vi "FTW-Collection-Construct-JSON.vi"(5 "Serialized Collection":string, 11 "error in":errorcluster) -> (4 "Collection":refnum<class "FTW-Collection.lvclass">, 6 "Valid Structure":bool, 15 "error out":errorcluster)   [LabVIEW 2012, in "FTW-Collection.lvclass"]
uses:
  FTW-Collection.lvclass
panel:
  # "Inputs"
  # "Outputs"
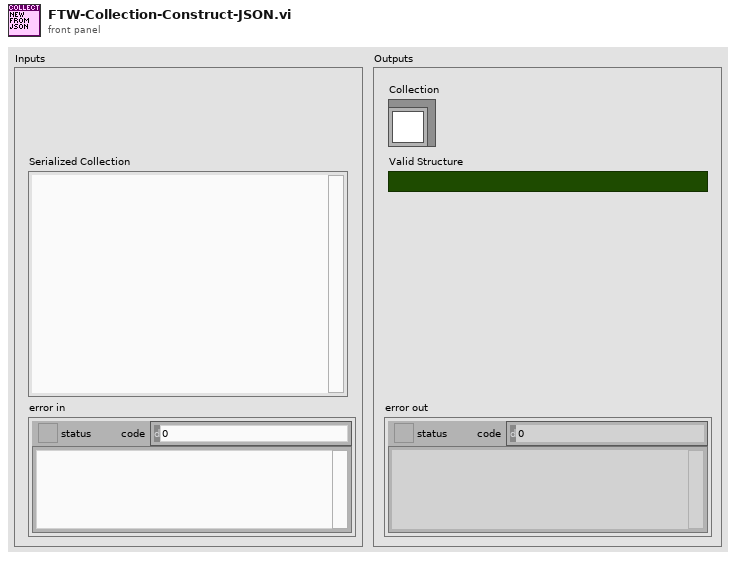
[diagram p1: front panel]
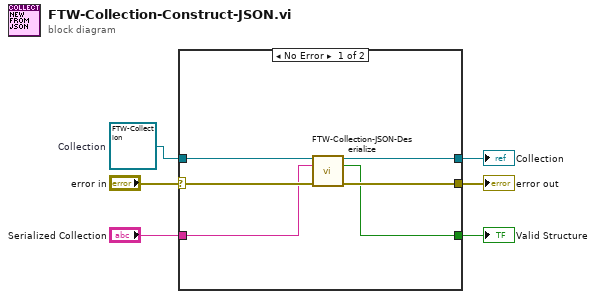
[diagram p0: block diagram]
diagram:
  w4 = refnum<class "FTW-Collection.lvclass"> refnum  # Collection
  n1 = case shown="No Error" "error in" {
    selector: "error in" -> [w11 w14]
    tunnel: [w9 w14] -> w6
    tunnel: w4 -> [w12 w13]
    tunnel: [w10 w13] -> w3
    tunnel: "Serialized Collection" -> [w8 _]
    tunnel: [w7 _] -> w1
    frame No Error {
      n2 = call "FTW-Collection-JSON-Deserialize.vi"("Collection"=w12, "Serialized Collection"=w8, "error in"=w11) -> ("Collection out"=w10:refnum<class "FTW-Collection.lvclass">, "Valid Structure"=w7:bool, "error out"=w9:errorcluster)  [unwired: 10 in]
    }
    frame Error {
    }
  }
  "error out" <- w6
  "Collection" <- w3
  "Valid Structure" <- w1
